vi "ESC control.vi"() -> ()   [LabVIEW 2015]
panel:
  out "Desired Position":dbl[](array[numeric])
  in  "Desired Orientation":dbl
  in  "Blimp Orientation":dbl
  in  "NAVIGATION STOP":bool
  out "Blimp Postion":dbl[](array[numeric])
  out "BLIMP POSITION":cluster{"Y":dbl[], "Y":dbl[]}[](graph)
  out "Chosen ESC(s)":string
  out "PWM Width":i32
  out "substring before match":string
  in  "String Input":string
  in  "SIMULATION STOP":bool
  # "ACTUAL STATES OF BLIMP"
  # "DESIRED STATES OF BLIMP"
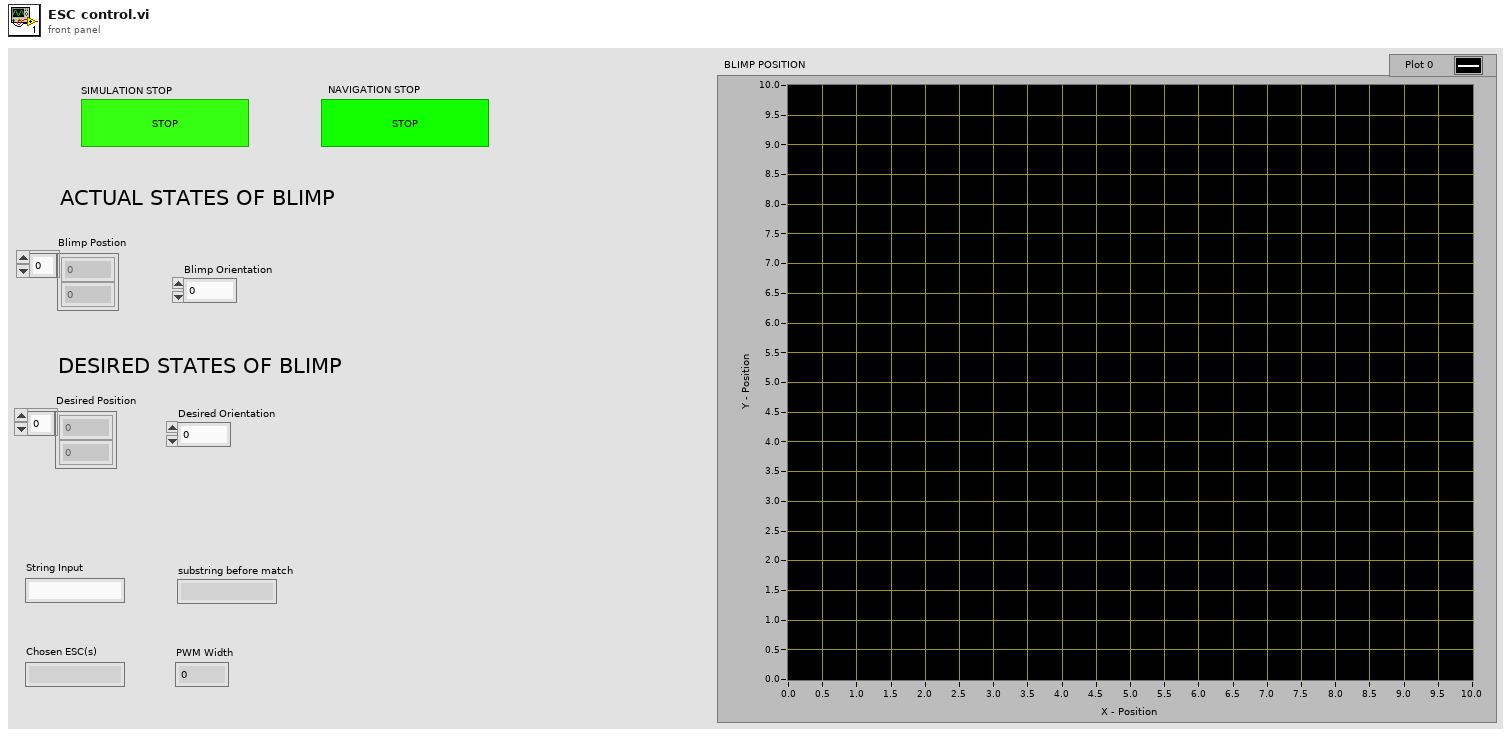
[diagram p1: front panel]
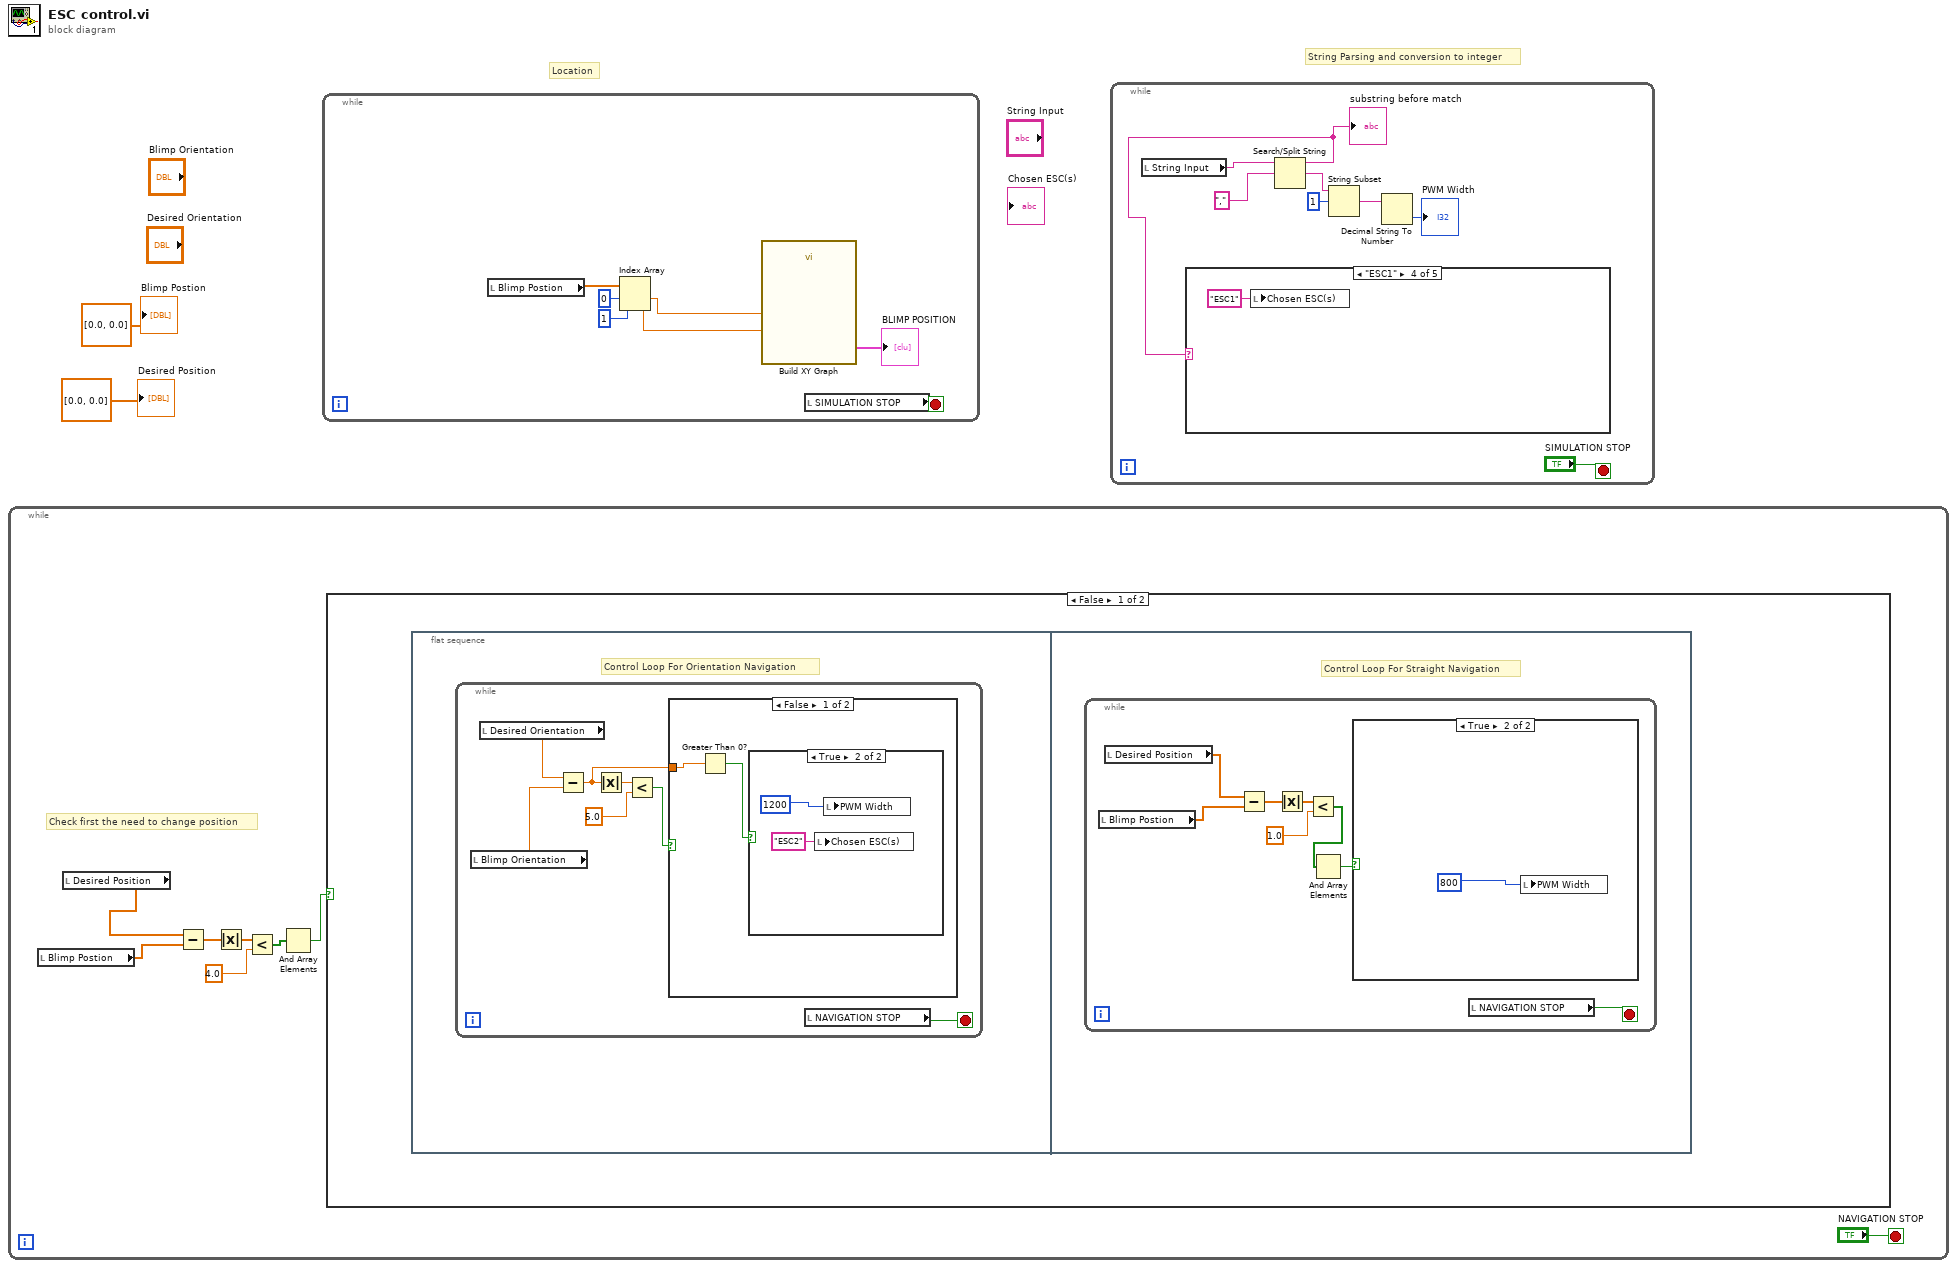
[diagram p0: block diagram]
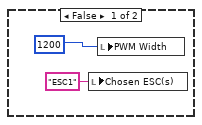
[diagram p2: hidden frame]
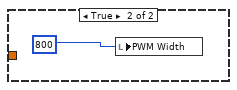
[diagram p3: hidden frame]
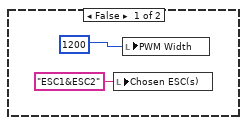
[diagram p4: hidden frame]
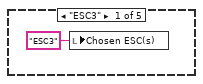
[diagram p6: hidden frame]
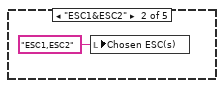
[diagram p7: hidden frame]
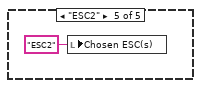
[diagram p9: hidden frame]
diagram:
  # "Location"
  # "String Parsing and conversion to integer"
  n1 = while {
    stop <- "NAVIGATION STOP" stop-if-true
    # "Check first the need to change position"
    n2 = local read "Blimp Postion"() -> (w6:dbl[])
    n3 = local read "Desired Position"() -> (w5:dbl[])
    n4 = Subtract(x=w5, y=w6) -> (x-y=w7:dbl[])
    n5 = Absolute Value(x=w7) -> (abs(x)=w8:dbl[])
    n6 = Less?(x=w8, y=4.0) -> (x < y?=w10:bool[])
    n7 = And Array Elements(Boolean array=w10) -> (logical AND=w4:bool)
    n8 = case shown="False" w4 {
      frame False {
        n9 = flat-sequence {
          frame #0 {
            # "Control Loop For Orientation Navigation"
            n10 = while {
              stop <- w13 stop-if-true
              n11 = local read "Blimp Orientation"() -> (w14:dbl)
              n12 = local read "Desired Orientation"() -> (w15:dbl)
              n13 = Subtract(x=w15, y=w14) -> (x-y=w12:dbl)
              n14 = Absolute Value(x=w12) -> (abs(x)=w16:dbl)
              n15 = Less?(x=w16, y=5.0) -> (x < y?=w11:bool)
              n16 = case shown="False" w11 {
                tunnel: w12 -> [w19 _]
                frame False {
                  n17 = Greater Than 0?(x=w19) -> (x > 0?=w18:bool)
                  n18 = case shown="True" w18 {
                    frame False {
                      n19 = local write "Chosen ESC(s)"("ESC1" ("Chosen ESC(s)")) -> ()
                      n20 = local write "PWM Width"(1200 ("PWM Width")) -> ()
                    }
                    frame True {
                      n21 = local write "Chosen ESC(s)"("ESC2" ("Chosen ESC(s)")) -> ()
                      n22 = local write "PWM Width"(1200 ("PWM Width")) -> ()
                    }
                  }
                }
                frame True {
                  n23 = local write "PWM Width"(800 ("PWM Width")) -> ()
                }
              }
              n24 = local read "NAVIGATION STOP"() -> (w13:bool)
            }
          }
          frame #1 {
            # "Control Loop For Straight Navigation"
            n25 = while {
              stop <- w25 stop-if-true
              n26 = local read "Blimp Postion"() -> (w32:dbl[])
              n27 = local read "Desired Position"() -> (w26:dbl[])
              n28 = Subtract(x=w26, y=w32) -> (x-y=w31:dbl[])
              n29 = Absolute Value(x=w31) -> (abs(x)=w30:dbl[])
              n30 = Less?(x=w30, y=1.0) -> (x < y?=w27:bool[])
              n31 = And Array Elements(Boolean array=w27) -> (logical AND=w28:bool)
              n32 = case shown="True" w28 {
                frame False {
                  n33 = local write "Chosen ESC(s)"("ESC1&ESC2" ("Chosen ESC(s)")) -> ()
                  n34 = local write "PWM Width"(1200 ("PWM Width")) -> ()
                }
                frame True {
                  n35 = local write "PWM Width"(800 ("PWM Width")) -> ()
                }
              }
              n36 = local read "NAVIGATION STOP"() -> (w25:bool)
            }
          }
        }
      }
      frame True {
      }
    }
  }
  n37 = while {
    stop <- w42 stop-if-true
    n38 = local read "Blimp Postion"() -> (w40:dbl[])
    n39 = Index Array(array=w40, index #1=0 ("index"), index #2=1 ("index")) -> (element #1=w37:dbl, element #2=w36:dbl)
    n40 = call "Build XY Graph"("Y Input"=w36, "X Input"=w37) -> ("XY Graph"=→"BLIMP POSITION":cluster{"Y":dbl[], "Y":dbl[]}[])  [unwired: 3 in, 6 out]
    n41 = local read "SIMULATION STOP"() -> (w42:bool)
  }
  n42 = while {
    stop <- "SIMULATION STOP" stop-if-true
    n43 = local read "String Input"() -> (w49:string)
    n44 = Search/Split String(string=w49, search string/char (-)=",") -> (substring before match=w43:string, match + rest of string=w47:string)  [unwired: 1 in, 1 out]
    "substring before match" <- w43
    n45 = case shown="\"ESC1\"" w43 {
      frame "ESC3" {
        n46 = local write "Chosen ESC(s)"("ESC3" ("Chosen ESC(s)")) -> ()
      }
      frame "ESC1&ESC2" {
        n47 = local write "Chosen ESC(s)"("ESC1,ESC2" ("Chosen ESC(s)")) -> ()
      }
      frame "Do Nothing", Default {
      }
      frame "ESC1" {
        n48 = local write "Chosen ESC(s)"("ESC1" ("Chosen ESC(s)")) -> ()
      }
      frame "ESC2" {
        n49 = local write "Chosen ESC(s)"("ESC2" ("Chosen ESC(s)")) -> ()
      }
    }
    n50 = String Subset(string=w47, offset (0)=1) -> (substring=w45:string)  [unwired: 1 in]
    n51 = Decimal String To Number(string=w45) -> (number=→"PWM Width":i32)  [unwired: 2 in, 1 out]
  }
  "Blimp Postion" <- dbl[] [0.0, 0.0] ("Blimp Postion")
  "Desired Position" <- dbl[] [0.0, 0.0] ("Blimp Postion")
